vi "Telemetry_engine.vi"(9 "Post dissable record time":dbl=10.0 format="%#_13g", 10 "Recording rate (Hz)":dbl=50.0 format="%#_13g", 11 "Telemetry data folder path":path) -> ()   [LabVIEW 2017, in "labview-standard-library.lvlib"]
uses:
  labview-standard-library.lvlib
  Telemetry_engine.ctl
  <vilib>/Rock Robotics/WPI/DriverStation/WPI_DriverStationRobotMode2.ctl
  <vilib>/Platform/TimedLoop/XDataNode/timing_clust.ctl
  <vilib>/Platform/TimedLoop/XDataNode/nitl_modes.ctl
  <vilib>/Platform/TimedLoop/XDataNode/wakeup.ctl
  system_tdms_write.vi
  dbl_tdms_write.vi
  bol_tdms_write.vi
  <vilib>/platform/TimedLoop/XDataNode/XDataNode.xnode
  <vilib>/Platform/TimedLoop/XDataNode/XDNodeRunTimeDep.lvlib
panel:
  in  "stop":bool
  out "Finished Late? [i-1]":bool
  out "error out":errorcluster
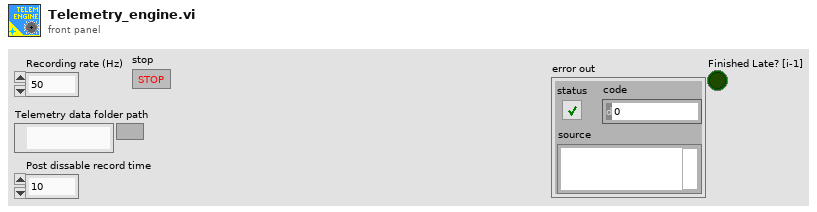
[diagram p1: front panel]
types:
  T1 = typedef "WPI_DriverStationRobotMode2.ctl" = enum16{"Autonomous Disabled", "Autonomous Enabled", "Teleop Disabled", "Teleop Enabled", "Disconnected", "Finish", "Test Disabled", "Test Enabled", "Emergency Stopped"}
  T2 = typedef "labview-standard-library.lvlib/Telemetry_engine.ctl" = enum16{"Wait", "Write"}
  T3 = typedef "XDNodeRunTimeDep.lvlib/timing_clust.ctl" = cluster{"Expected End [f-1]":u64, "Actual End [f-1]":u64, "Finished Late? [f-1]":bool, "Expected End [i-1]":u64, "Actual End [i-1]":u64, "Finished Late? [i-1]":bool, "Expected Start [i]":u64, "Actual Start [i]":u64, "Expected Start [f]":u64, "Actual Start [f]":u64, "Source Name":string, "Structure Name":string, "Period":i64, "Deadline":i64, "Offset":i64, "Start":i64, "Priority":i32, "Timeout":i32, "Mode":T4, "Wakeup Reason":T5, "Error":errorcluster, "Source Type":string, "Secondary Source Type":string, "Global End Time":u64, "Global Start Time":u64, "Frame Duration":u64, "Iteration Duration":u64, "Assigned CPU":i32, "I/O Scan Engine Mode":u32}
  T4 = typedef "XDNodeRunTimeDep.lvlib/nitl_modes.ctl" = enum32{"No Change", "Process missed periods, maintain original phase", "Discard missed periods, maintain original phase", "Process missed periods, ignore original phase", "Discard missed periods, ignore original phase"}
  T5 = typedef "XDNodeRunTimeDep.lvlib/wakeup.ctl" = enum32{"Normal", "Aborted", "Asynchronous wakeup", "Timing source error", "Timed loop error", "Timeout"}
  T6 = typedef "labview-standard-library.lvlib/Channel&data_arrays.ctl" = cluster{"Subsystem name arrays":string[], "DBL Data arrays":dbl[][][], "BOL Data arrays":bool[][][], "BOL channel name arrays":string[][], "DBL channel name arrays":string[][]}
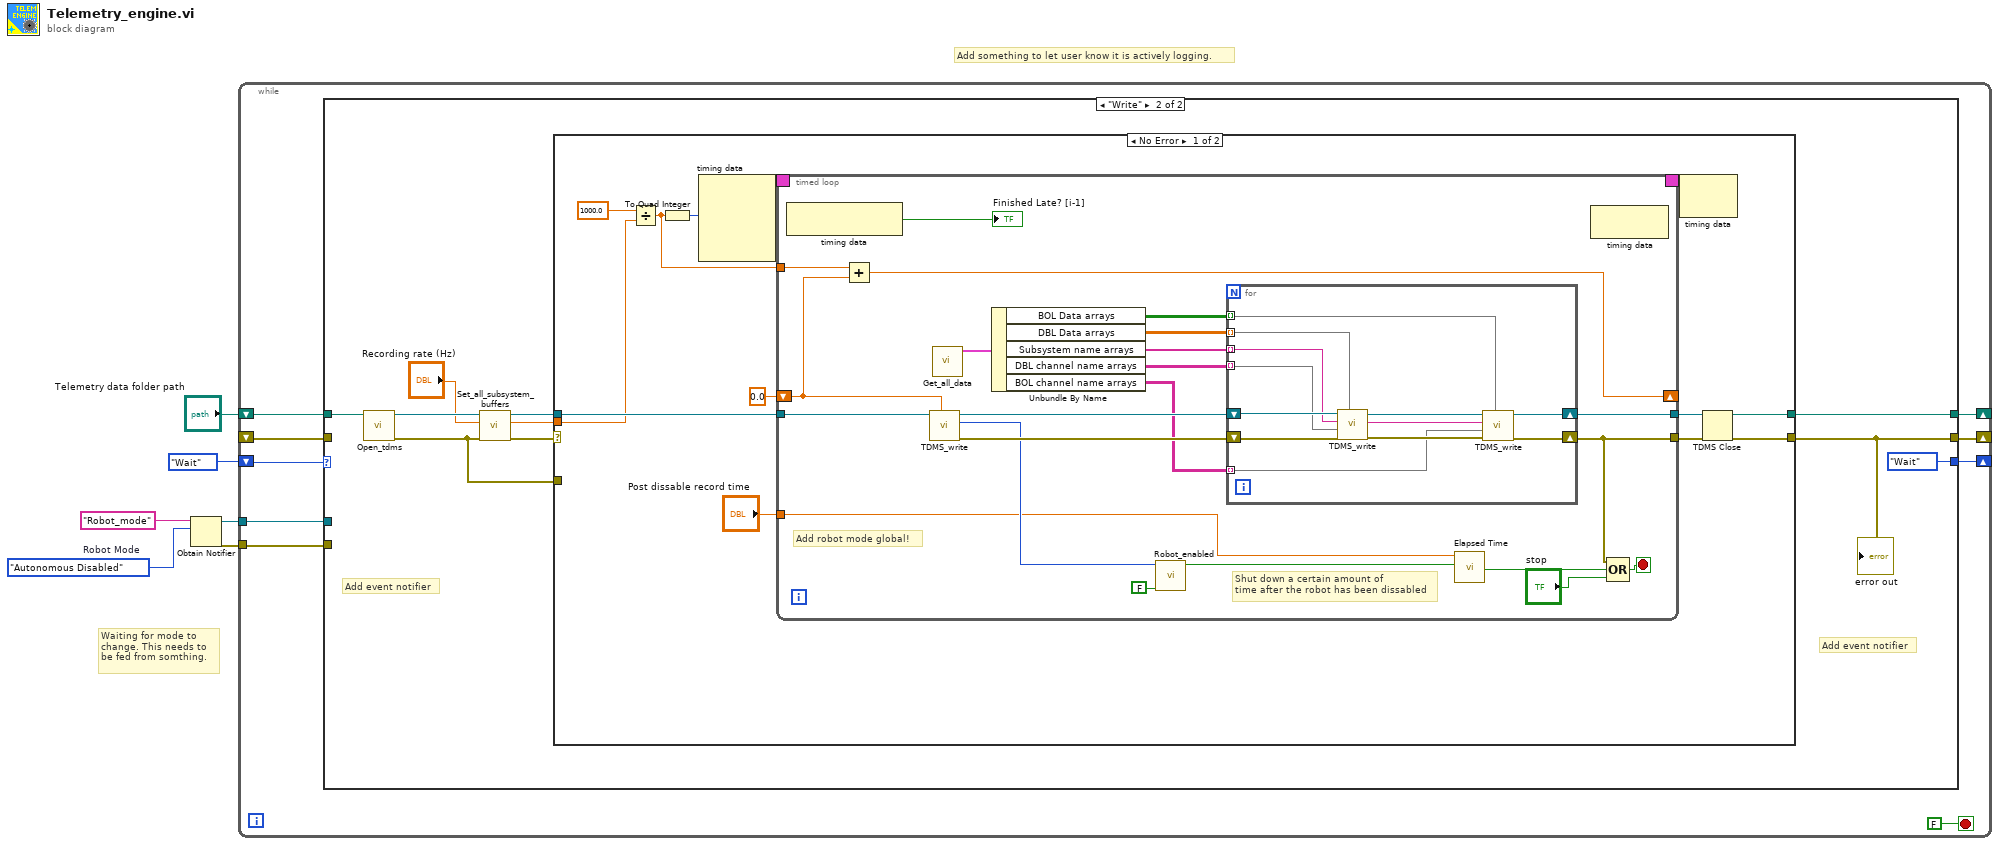
[diagram p0: block diagram]
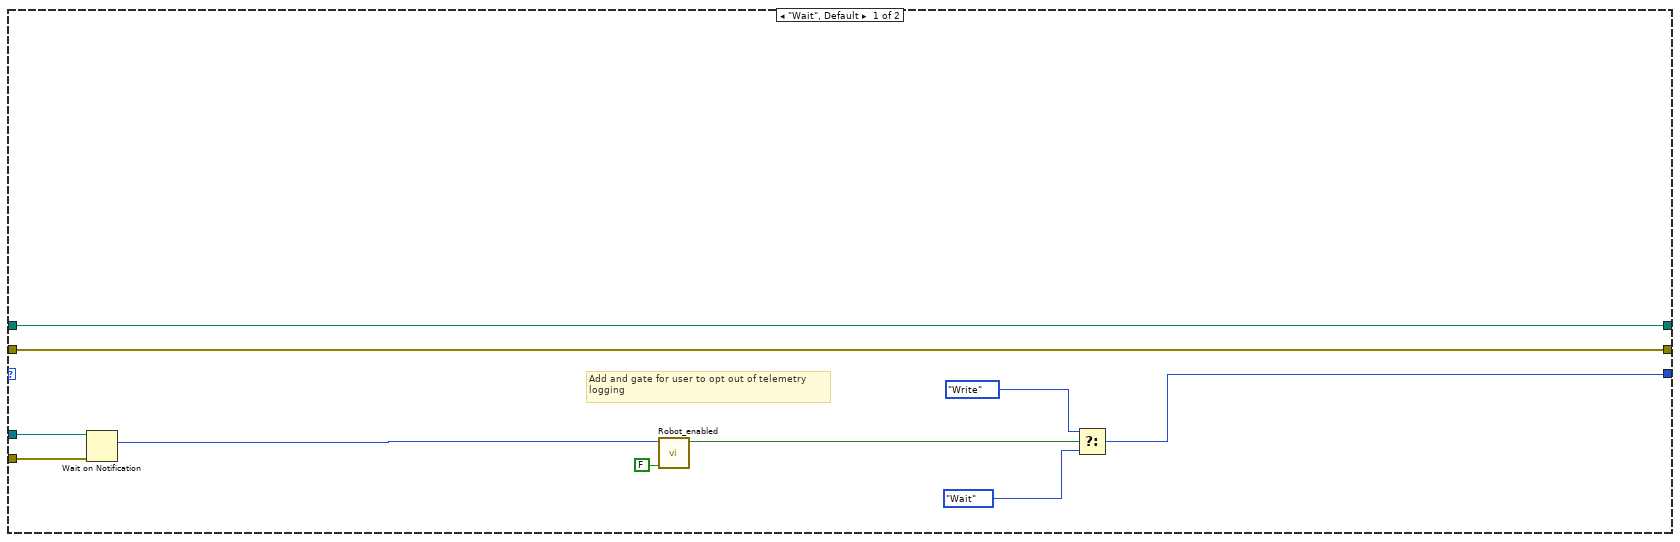
[diagram p2: hidden frame]
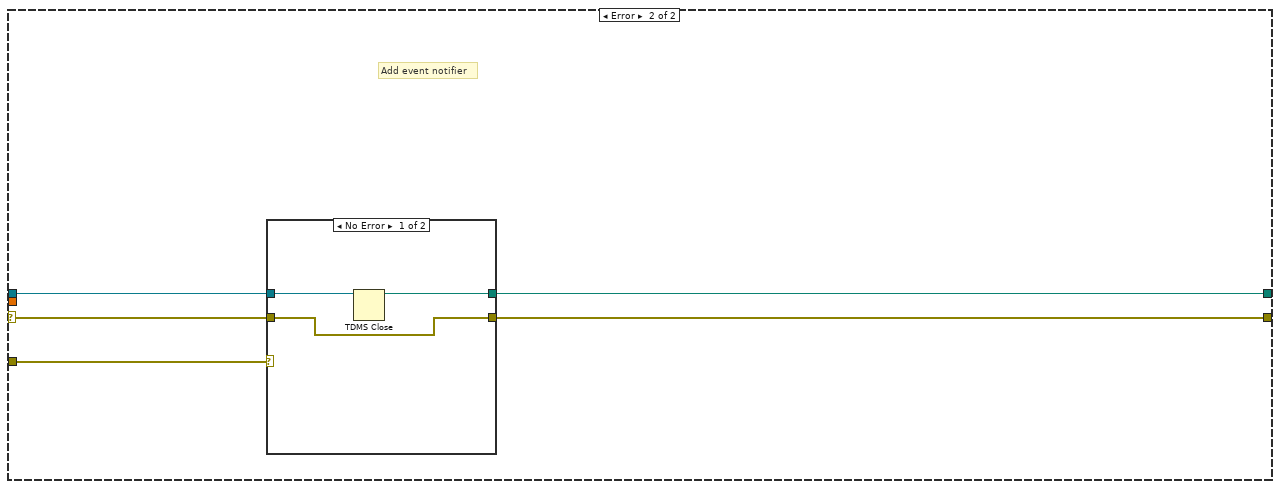
[diagram p3: hidden frame]
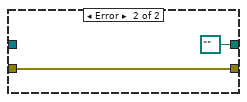
[diagram p4: hidden frame]
diagram:
  w2 = WPI_DriverStationRobotMode2."Autonomous Disabled"  # Robot Mode
  # "Waiting for mode to\nchange. This needs to\nbe fed from somthing."
  # "Add something to let user know it is actively logging."
  n1 = Obtain Notifier(name (unnamed)="Robot_mode", notification data type=w2) -> (notifier out=w4:refnum<notifier>, error out=w3:errorcluster)  [unwired: 2 in, 1 out]
  n2 = while {
    shift-right: [w13] -> _
    shift-left: "Telemetry data folder path" -> [w14]
    shift-right: [w12] -> _
    shift-left: _ -> [w11]
    shift-right: [w9] -> _
    shift-left: Telemetry_engine."Wait" -> [w10]
    tunnel: w4 -> [w8]
    tunnel: w3 -> [w7]
    stop <- FALSE stop-if-true
    n3 = case shown="\"Write\"" w10 {
      tunnel: w14 -> [w24 w31]
      tunnel: [w24 w30] -> w13
      tunnel: [w25 w29] -> w12
      tunnel: w11 -> [w25 _]
      tunnel: [w23 Telemetry_engine."Wait"] -> w9
      tunnel: w8 -> [w18 _]
      tunnel: w7 -> [w16 _]
      frame "Wait", Default {
        # "Add and gate for user to opt out of telemetry \nlogging"
        n4 = Wait on Notification(notifier=w18, error in (no error)=w16) -> (notification=w17:T1)  [unwired: 2 in, 3 out]
        n5 = call "Robot_enabled.vi"("Include test mode? (F)"=FALSE, "Robot Mode in"=w17) -> ("Enabled?"=w20:bool)  [unwired: 9 in]
        n6 = Select(t=Telemetry_engine."Write", s=w20, f=Telemetry_engine."Wait") -> (s? t:f=w23:T2)
      }
      frame "Write" {
        # "Add event notifier"
        # "Add event notifier"
        n7 = call "Open_tdms.vi"("Folder path"=w31) -> ("error out"=w26:errorcluster, "tdms refnum out"=w34:refnum<k34>)  [unwired: 8 in, 1 out]
        n8 = call "Set_all_subsystem_buffers.vi"("error in"=w26, "Record rate (Hz)"="Recording rate (Hz)", "Refnum in"=w34) -> ("error out"=w27:errorcluster, "Refnum out"=w33:refnum<k34>)  [unwired: 7 in]
        n9 = case shown="No Error" w27 {
          selector: w27 -> [_ w93]
          tunnel: w33 -> [w45 w90]
          tunnel: "Recording rate (Hz)" -> [w43 _]
          tunnel: [w42 w89] -> w30
          tunnel: [w39 w92] -> w29
          tunnel: w26 -> [_ w91]
          frame No Error {
            n10 = Divide(x=1000.0, y=w43) -> (x/y=w35:dbl)
            n11 = To Quad Integer(1:w35) -> (0:w37:i64)
            n12 = node-c288(w37) -> (w47:T3)  [unwired: 3 in]
            n13 = timed-loop {
              tunnel: w45 -> [w67]
              tunnel: [w63] -> w41
              tunnel: [w61] -> w40
              tunnel: "Post dissable record time" -> [w60]
              timing: w47 -> [_]
              timing-out: [_] -> w46
              shift-right: [w57] -> _
              shift-left: 0.0 -> [w59]
              tunnel: w35 -> [w58]
              stop <- w62 stop-if-true
              # "Shut down a certain amount of\ntime after the robot has been dissabled"
              # "Add robot mode global!"
              n14 = node-c288() -> (→"Finished Late? [i-1]":bool)  [unwired: 1 in]
              n15 = Add(x=w58, y=w59) -> (x+y=w57:dbl)
              n16 = call-poly "TDMS_write.vi"("Timer in"=w59, "tdms refnum in"=w67) -> ("error out"=w68:errorcluster, "Robot Mode out"=w66:T1, "tdms refnum out"=w69:refnum<k34>)  [unwired: 7 in]
              n17 = call "Get_all_data.vi"() -> ("Channel & data arrays out"=w50:T6)  [unwired: 10 in, 1 out]
              n18 = Unbundle By Name(w50) -> ("BOL Data arrays"=w55:bool[][][], "DBL Data arrays"=w54:dbl[][][], "Subsystem name arrays"=w53:string[], "DBL channel name arrays"=w52:string[][], "BOL channel name arrays"=w51:string[][])
              n19 = call "Robot_enabled.vi"("Include test mode? (F)"=FALSE, "Robot Mode in"=w66) -> ("Enabled?"=w65:bool)  [unwired: 9 in]
              n20 = for {
                shift-right: [w83] -> w61
                shift-left: w68 -> [w82]
                shift-right: [w81] -> w63
                shift-left: w69 -> [w79]
                tunnel: w52 -> [w77] mode=indexing
                tunnel: w53 -> [w76] mode=indexing
                tunnel: w51 -> [w75] mode=indexing
                tunnel: w54 -> [w74] mode=indexing
                tunnel: w55 -> [w73] mode=indexing
                n21 = call-poly "TDMS_write.vi"("DBL Data in"=w74, "error in (no error)"=w82, "channel name(s) in"=w77, "Subsystem name in"=w76, "tdms file"=w79) -> ("error out"=w84:errorcluster, "Subsystem name out"=w78:string, "tdms file out"=w80:refnum<k34>)  [unwired: 4 in]
                n22 = call-poly "TDMS_write.vi"("Boolean Data in"=w73, "error in (no error)"=w84, "channel name(s) in"=w75, "Subsystem name in"=w78, "tdms file"=w80) -> ("error out"=w83:errorcluster, "tdms file out"=w81:refnum<k34>)  [unwired: 4 in, 1 out]
              }
              n23 = call "Elapsed Time"("Time Target (s)"=w60, "Reset"=w65) -> ("Time has Elapsed"=w64:bool)  [unwired: 10 in, 7 out]
              n24 = node-c288() -> ()  [unwired: 1 in, 1 out]
              n25 = Compound Arithmetic op=OR(w61, w64, "stop") -> (w62:bool)
            }
            n26 = node-c288(w46) -> ()  [unwired: 1 out]
            n27 = TDMS Close(8:w40, 11:w41) -> (0:w39:errorcluster, 3:w42:path)
          }
          frame Error {
            # "Add event notifier"
            n28 = case shown="No Error" w91 {
              tunnel: [w94 w98] -> w92
              tunnel: w93 -> [w94 w98]
              tunnel: w90 -> [w96 _]
              tunnel: [w95 path "" ("file path out")] -> w89
              frame No Error {
                n29 = TDMS Close(11:w96) -> (3:w95:path)  [unwired: 1 in, 1 out]
              }
              frame Error {
              }
            }
          }
        }
        "error out" <- w29
      }
    }
  }
